vi "NI 直方圖、灰階像素強度.vi"() -> ()   [LabVIEW 2019]
panel:
  out "Line Profile (Line Profile 1)":u8[][](array[numeric])
  out "Histogram (Histogram 1)":u32[][](array[numeric])
  in  "stop":bool
  out "Image":T1(plugin-control)
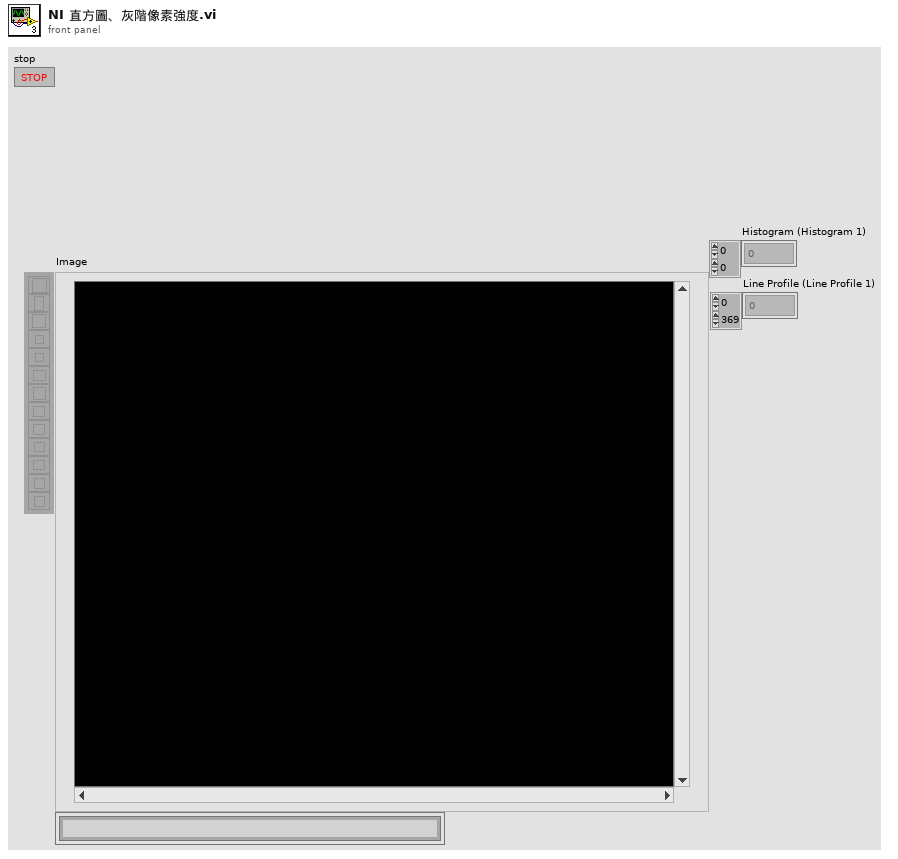
[diagram p1: front panel]
types:
  T1 = typedef "IMAQ Image.ctl" = refnum<image>
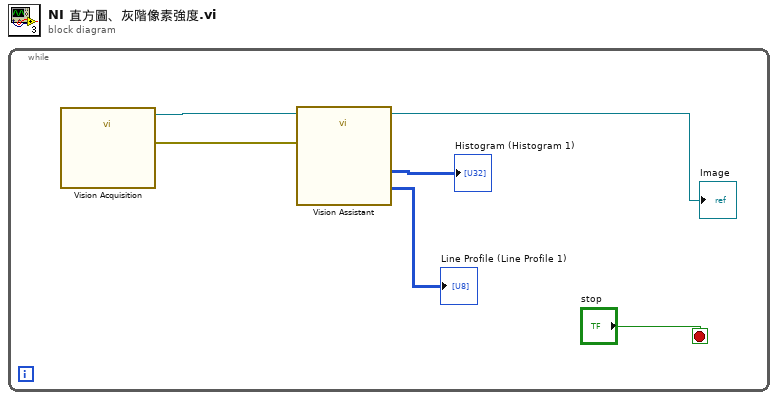
[diagram p0: block diagram]
diagram:
  n1 = while {
    stop <- "stop" stop-if-true
    n2 = call "Vision Acquisition"() -> ("Image Out"=w6:T1, "error out"=w5:errorcluster)  [unwired: 25 in, 1 out]
    n3 = call "Vision Assistant"("Image In"=w6, "error in"=w5) -> ("Image Out"=→"Image":T1, "Histogram (Histogram 1)"=→"Histogram (Histogram 1)":u32[][], "Line Profile (Line Profile 1)"=→"Line Profile (Line Profile 1)":u8[][])  [unwired: 22 in, 1 out]
  }
